vi "CoPilotControlFlow.vi"() -> (1 "Arm Shoulder Control":dbl, 2 "Arm Base Control":dbl, 3 "Pneumatic Control":dbl)   [LabVIEW 2017]
uses:
  <vilib>/Rock Robotics/WPI/Utilities/WPI_GetSetVariantRefNum.vi
panel:
  out "Buttons":bool[](array[boolean])
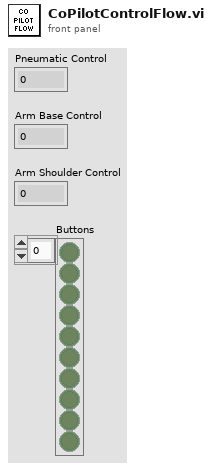
[diagram p1: front panel]
types:
  T1 = typedef "WPI_JoystickDevRef.ctl" = cluster{"Device":T2}
  T2 = typedef "WPI_JoystickDeviceEnum.ctl" = enum16{"USB 0", "USB 1", "USB 2", "USB 3", "USB 4", "USB 5"}
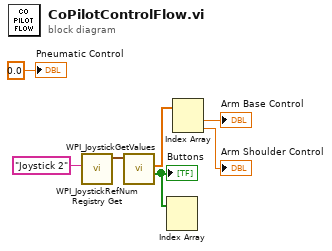
[diagram p0: block diagram]
diagram:
  n1 = call <vilib>:"WPI_JoystickRefNum Registry Get.vi"("refnum name"="Joystick 2") -> ("JoystickDevRef"=w3:T1)  [unwired: 1 in, 9 out]
  n2 = call <vilib>:"WPI_JoystickGetValues.vi"("JoystickDevRef"=w3) -> ("Buttons"=w5:bool[], "Axes"=w4:dbl[])  [unwired: 6 in, 3 out]
  "Buttons" <- w5
  n3 = Index Array(array=w5) -> ()  [unwired: 2 in, 2 out]
  n4 = Index Array(array=w4) -> (element #1=→"Arm Base Control":dbl, element #2=→"Arm Shoulder Control":dbl)  [unwired: 2 in]
  "Pneumatic Control" <- 0.0 ("Pneumatic Control")
